vi "sort resource entries.vi"(7 "Sort Type":T1 items=["RIO device", "resource", "input type", "datatype", "reserver"], 8 "error in (no error)":errorcluster, 11 "resource table in":string[][](array[string])) -> (0 "error out":errorcluster, 3 "resource table out":string[][](array[string]))   [LabVIEW 2016, in "FPGA Resource Manager.lvlib"]
uses:
  FPGA Resource Manager.lvlib
  viz_type.ctl
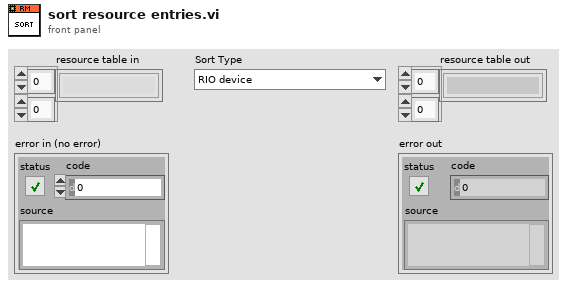
[diagram p1: front panel]
types:
  T1 = typedef "FPGA Resource Manager.lvlib/viz_type.ctl" = u16
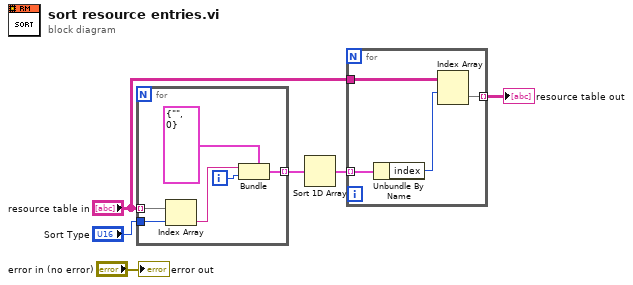
[diagram p0: block diagram]
diagram:
  n1 = for {
    tunnel: "resource table in" -> [w9] mode=indexing
    tunnel: "Sort Type" -> [w8]
    tunnel: [w11] -> w5 mode=indexing
    i -> [w12]
    n2 = Index Array(array=w9, index=w8) -> (element=w7:string)
    n3 = Bundle(cluster=cluster{"key":string, "index":i32} {"key"="", "index"=0}, "key"=w7, "index"=w12) -> (w11:cluster{"key":string, "index":i32})
  }
  n4 = Sort 1D Array(array=w5) -> (sorted array=w4:cluster{"key":string, "index":i32}[])
  n5 = for {
    tunnel: w4 -> [w16] mode=indexing
    tunnel: "resource table in" -> [w15]
    tunnel: [w13] -> w2 mode=indexing
    n6 = Unbundle By Name(w16) -> ("index"=w14:i32)
    n7 = Index Array(array=w15, index (row)=w14) -> (element=w13:string[])  [unwired: 1 in]
  }
  "resource table out" <- w2
  "error out" <- "error in (no error)"
